vi "Custom label Print.vi"() -> ()   [LabVIEW 2014]
panel:
  out "EOL Stations":string
  out "OEM":string
  out "VISA资源名称":refnum<visa-resource-name>="PrintGK420T_ST30"
  in  "停止":bool
  out "error out":errorcluster
  out "Ser nr":string
  out "IRS nr":string
  in  "簇":T1
  # "标签预览"
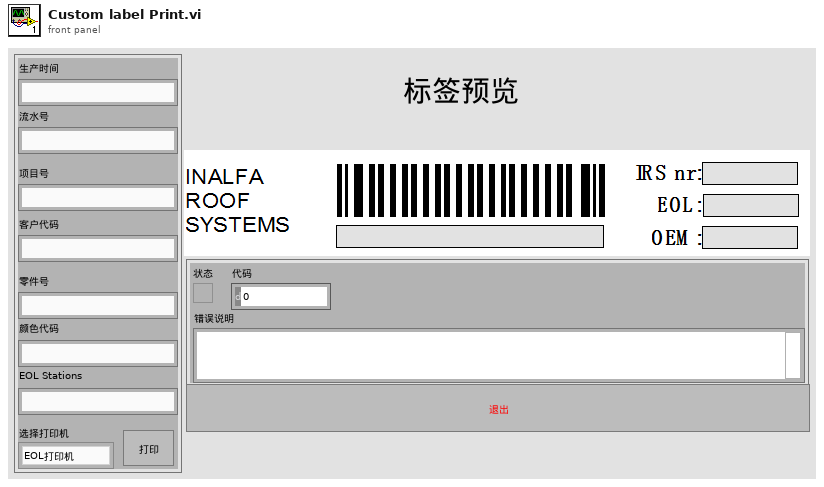
[diagram p1: front panel]
types:
  T1 = cluster{"生产时间":string, "流水号":string, "项目号":string, "客户代码":string, "零件号":string, "选择打印机":enum16{"EOL打印机", "打凹点打印机"}, "打印":bool, "颜色代码":string, "EOL Stations":string}
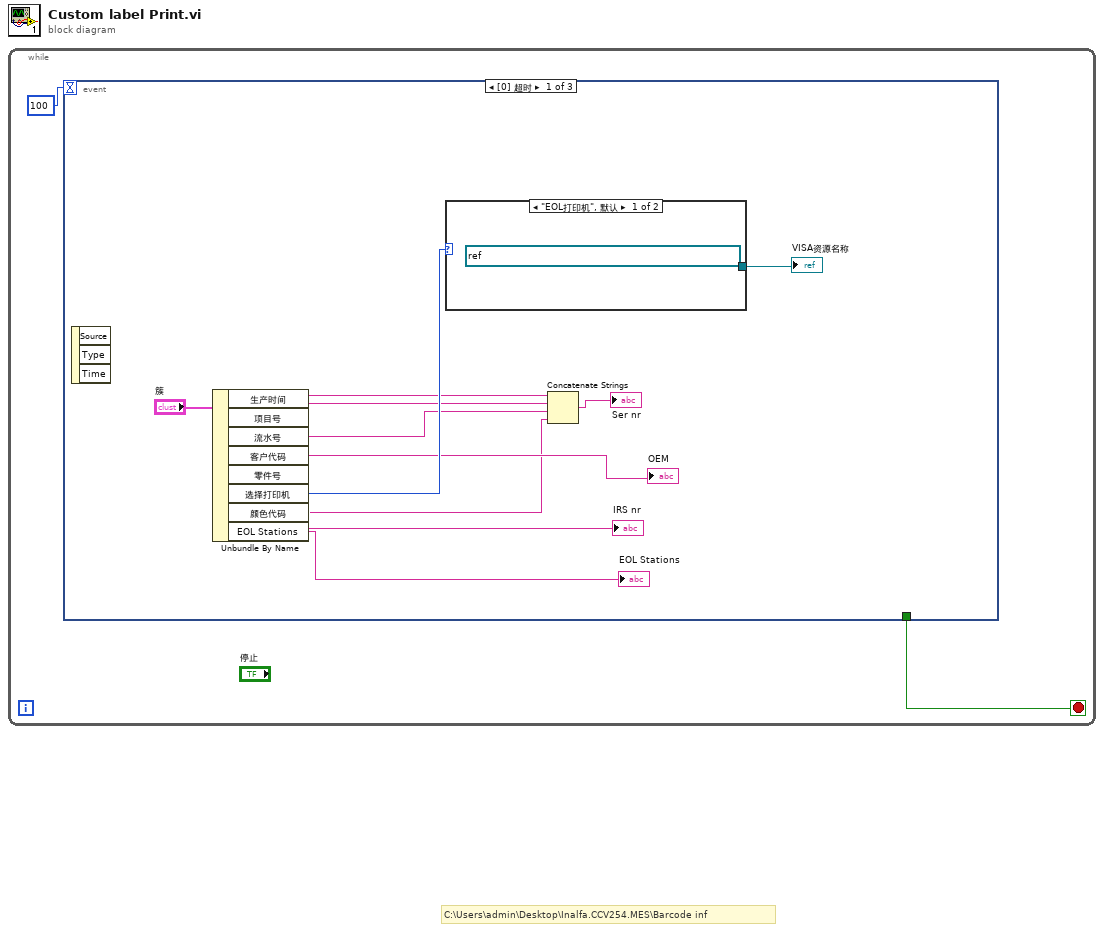
[diagram p0: block diagram]
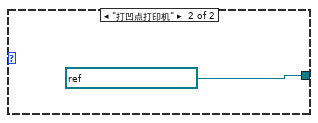
[diagram p2: hidden frame]
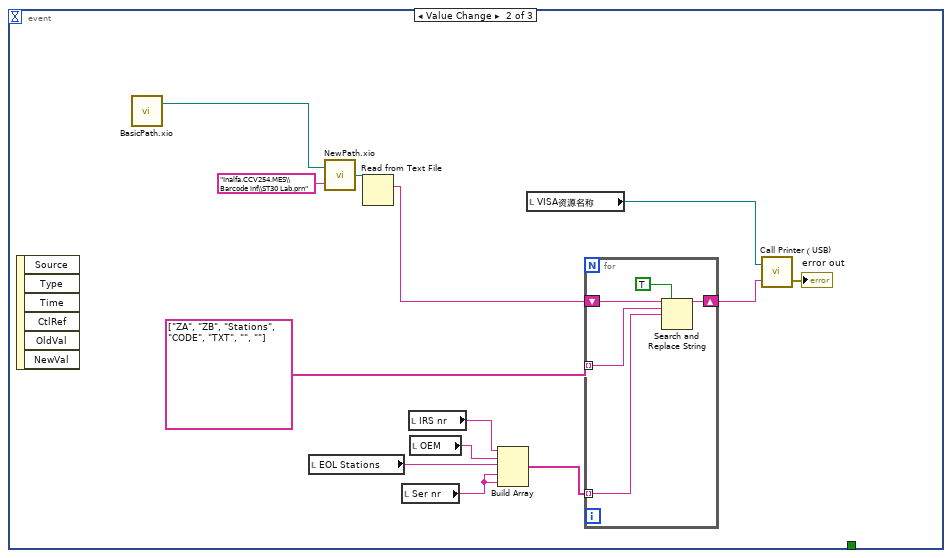
[diagram p3: hidden frame]
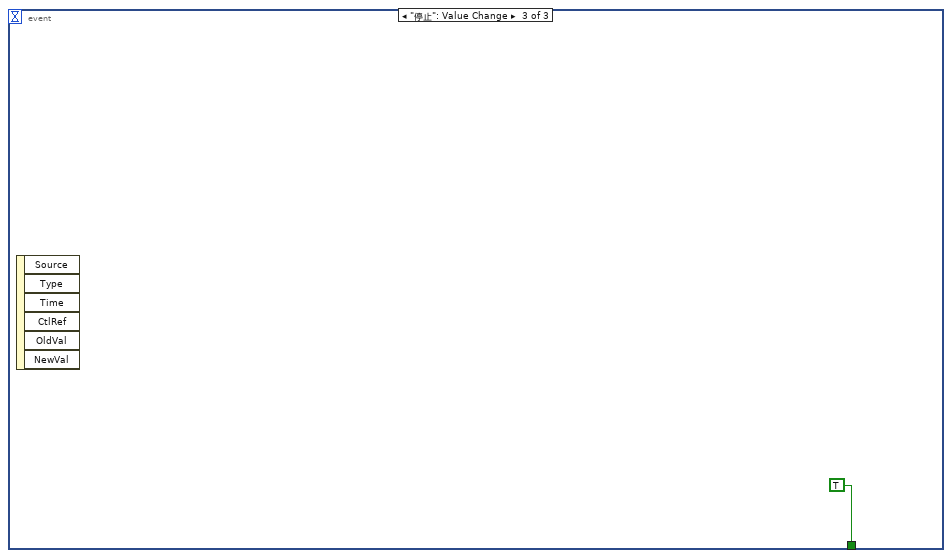
[diagram p4: hidden frame]
diagram:
  # "C:\\Users\\admin\\Desktop\\Inalfa.CCV254.MES\\Barcode inf"
  n1 = while {
    stop <- w2 stop-if-true
    n2 = event shown="[0] 超时" {
      selector: _ -> [_ _ _]
      dyn-events: _ -> [_ _ _]
      timeout: 100 -> [_ _ _]
      tunnel: [_ _ TRUE] -> w2
      event Timeout {
        n3 = event-data() -> ()  [unwired: 1 in, 3 out]
        n4 = Unbundle By Name("簇") -> ("生产时间"=w10:string, "项目号"=w6:string, "流水号"=w5:string, "客户代码"=→"OEM":string, "零件号"=→"IRS nr":string, "选择打印机"=w12:enum16{"EOL打印机", "打凹点打印机"}, "颜色代码"=w4:string, "EOL Stations"=→"EOL Stations":string)
        n5 = case shown="\"EOL打印机\", 默认" w12 {
          tunnel: [refnum<visa-resource-name> "USB0::0x0A5F::0x0081::29J194401307::RAW" ("VISA资源名称") refnum<visa-resource-name> "PrintGK420T_ST90" ("VISA资源名称")] -> w11
          frame "EOL打印机", Default {
          }
          frame "打凹点打印机" {
          }
        }
        "VISA资源名称" <- w11
        n6 = Concatenate Strings(w10, w6, w5, w4) -> (→"Ser nr":string)
      }
      event "簇.打印": Value Change {
        n7 = event-data() -> ()  [unwired: 1 in, 6 out]
        n8 = call "BasicPath.xio.vi"() -> ("stripped path"=w18:path)  [unwired: 1 in, 1 out]
        n9 = local read "EOL Stations"() -> (w21:string)
        n10 = call "NewPath.xio.vi"("Append path"="Inalfa.CCV254.MES\\Barcode inf\\ST30 Lab.prn", "Basic path"=w18) -> ("New path"=w16:path)
        n11 = Read from Text File(file (use dialog)=w16) -> (text=w27:string)  [unwired: 3 in, 3 out]
        n12 = local read "Ser nr"() -> (w20:string)
        n13 = local read "IRS nr"() -> (w22:string)
        n14 = local read "OEM"() -> (w23:string)
        n15 = Build Array(w22, w23, w21, w20, w20) -> (w26:string[])
        n16 = local read "VISA资源名称"() -> (w24:refnum<visa-resource-name>)
        n17 = for {
          tunnel: string[] ["ZA", "ZB", "Stations", "CODE", "TXT", "", ""] -> [w33] mode=indexing
          shift-right: [w31] -> w25
          shift-left: w27 -> [w32]
          tunnel: w26 -> [w30] mode=indexing
          n18 = Search and Replace String(replace all?=TRUE ("替换全部？(F)"), input string=w32, search string=w33, replace string=w30) -> (result string=w31:string)  [unwired: 4 in, 3 out]
        }
        n19 = call "Call Printer（USB).vi"("写入缓冲区"=w25, "VISA资源名称"=w24) -> ("error out"=→"error out":errorcluster)  [unwired: 1 out]
      }
      event "停止": Value Change {
        n20 = event-data() -> ()  [unwired: 1 in, 6 out]
      }
    }
  }
